vi "exp 9 imaq and vision.vi"() -> ()   [LabVIEW 2025]
panel:
  in  "Use File Path Image Type":bool=TRUE
  out "Image":T1(plugin-control)
  in  "File Path":path
  in  "Image Type":T2 items=["Grayscale (U8)", "Grayscale (I16)", "Grayscale (SGL)", "Complex (CSG)", "RGB (U32)", "HSL (U32)", "RGB (U64)", "Grayscale (U16)"]
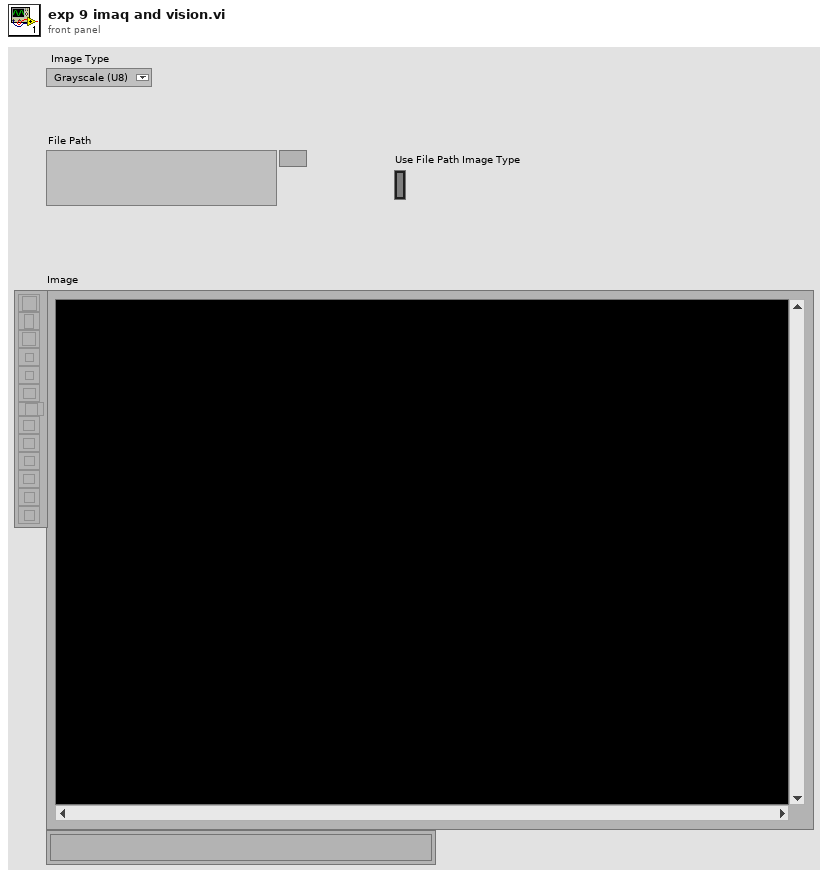
[diagram p1: front panel]
types:
  T1 = typedef "IMAQ Image.ctl" = refnum<image>
  T2 = typedef "Image Type" = u32
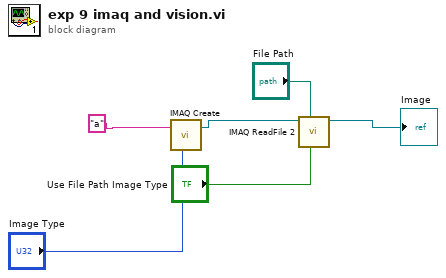
[diagram p0: block diagram]
diagram:
  n1 = call "IMAQ Create"("Image Name"="a", "Image Type"="Image Type") -> ("New Image"=w4:T1)  [unwired: 3 in, 1 out]
  n2 = call "IMAQ ReadFile 2"("Use File Path Image Type"="Use File Path Image Type", "File Path"="File Path", "Image"=w4) -> ("Image Out"=→"Image":T1)  [unwired: 4 in, 4 out]
